vi "Fit Real Lorentzian.vi"(7 "Initial guess":T1={"Amplitude"=1000.0, "Center"=694.3, "Width"=0.4} {"Width" format="%#_gnm"; "Center" format="%#_gnm"}, 8 "Error In":errorcluster, 10 "X":dbl[](array[numeric]), 11 "Y":dbl[](array[numeric])) -> (0 "Error Out":errorcluster, 5 "Fit":T1={"Amplitude"=1000.0, "Center"=694.3, "Width"=0.4} {"Width" format="%#_gnm"; "Center" format="%#_gnm"})   [LabVIEW 2016]
uses:
  Peak Parameters.ctl
  <vilib>/gmath/NumericalOptimization/Nonlinear Curve Fit LM bound.vi
  <vilib>/gmath/NI_Gmath.lvlib
panel:
  out "number of function calls":i32
  out "XY Graph":cluster{"all rows":dbl[], "Data out":dbl[]}[](graph)
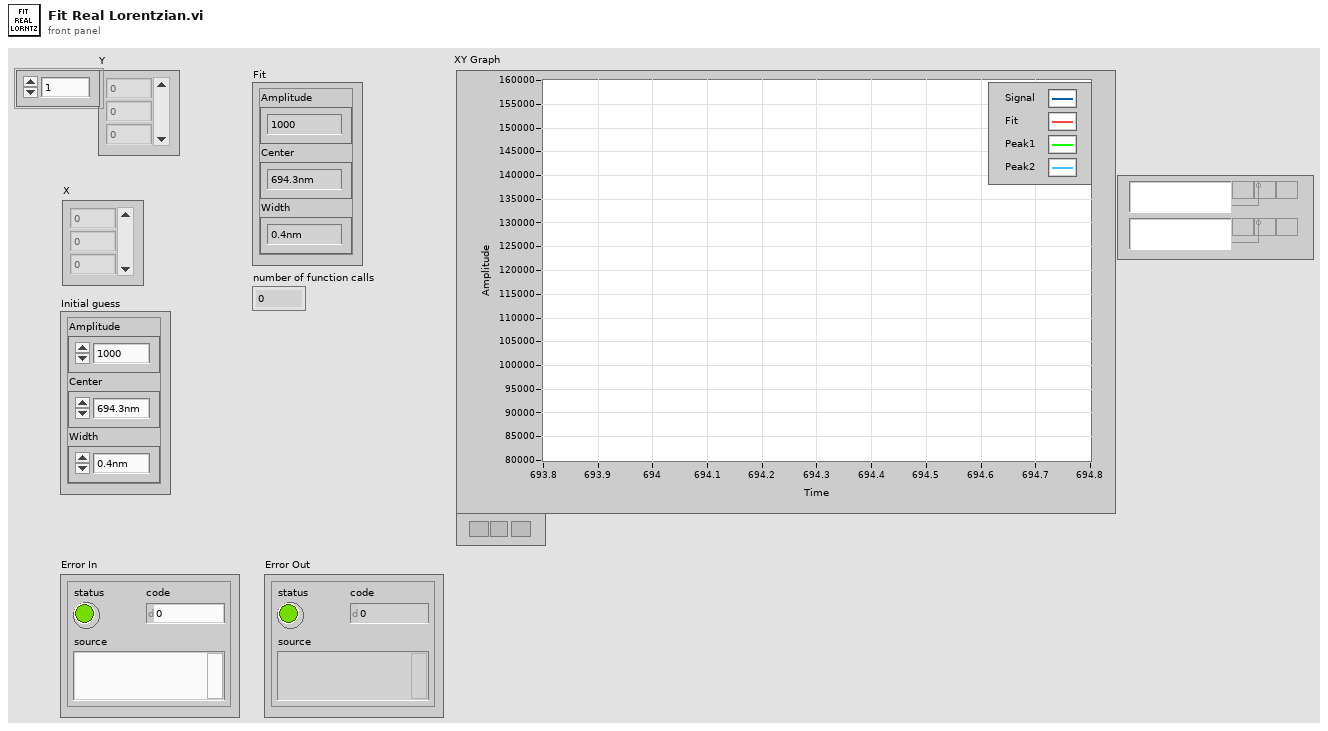
[diagram p1: front panel]
types:
  T1 = typedef "Peak Parameters.ctl" = cluster{"Amplitude":dbl, "Center":dbl, "Width":dbl}
  T2 = cluster{"parameter minimum":dbl[], "parameter maximum":dbl[]}
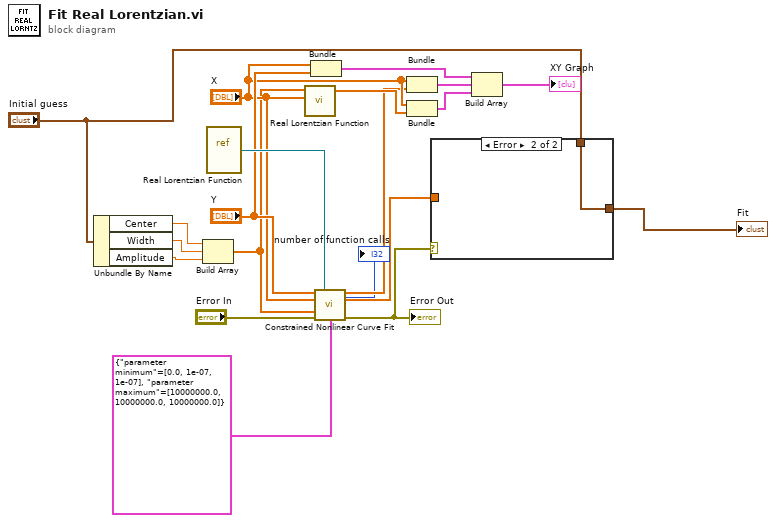
[diagram p0: block diagram]
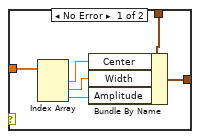
[diagram p2: hidden frame]
diagram:
  n1 = Unbundle By Name("Initial guess") -> ("Center"=w20:dbl, "Width"=w19:dbl, "Amplitude"=w16:dbl)
  n2 = Build Array(w20, w19, w16) -> (w5:dbl[])
  n3 = vi-ref "Real Lorentzian Function.vi"() -> (w18:refnum<vi>)
  n4 = call "Real Lorentzian Function.vi"("X"="X", "a"=w5) -> ("f(X,a)"=w10:dbl[])  [unwired: 2 in, 2 out]
  n5 = Bundle("X"="X", "Y"="Y") -> (w13:cluster{"X":dbl[], "Y":dbl[]})  [unwired: 1 in]
  n6 = call-poly <vilib>:"Constrained Nonlinear Curve Fit.vi"("Y"="Y", "f(x,a)"=w18, "X"="X", "initial parameters"=w5, "error in (no error)"="Error In", "parameter bounds"=T2 {"parameter minimum"=[0.0, 1e-07, 1e-07], "parameter maximum"=[10000000.0, 10000000.0, 10000000.0]}) -> ("number of function calls"=→"number of function calls":i32, "best nonlinear fit"=w4:dbl[], "best fit parameters"=w15:dbl[], "error out"=w2:errorcluster)  [unwired: 4 in, 2 out]
  "Error Out" <- w2
  n7 = Bundle("X"="X", "best nonlinear fit"=w4) -> (w12:cluster{"X":dbl[], "best nonlinear fit":dbl[]})  [unwired: 1 in]
  n8 = Bundle("X"="X", "f(X,a)"=w10) -> (w9:cluster{"X":dbl[], "f(X,a)":dbl[]})  [unwired: 1 in]
  n9 = case shown="Error" w2 {
    tunnel: "Initial guess" -> [w26 w27]
    tunnel: w15 -> [w25 _]
    tunnel: [w21 w27] -> w14
    frame No Error {
      n10 = Index Array(array=w25) -> (element #1=w24:dbl, element #2=w23:dbl, element #3=w22:dbl)  [unwired: 3 in]
      n11 = Bundle By Name(cluster=w26, "Center"=w24, "Width"=w23, "Amplitude"=w22) -> (w21:T1)
    }
    frame Error {
    }
  }
  "Fit" <- w14
  n12 = Build Array(w13, w12, w9) -> (→"XY Graph":cluster{"X":dbl[], "f(X,a)":dbl[]}[])
